vi "Configure Threshold Range.vi"(6 "Auto Threshold Range (T: Enable)":bool=TRUE, 7 "Range (10)":dbl=10.0, 8 "error in (no error)":errorcluster, 9 "Channel List(\"\")":string, 10 "Function (10:Frequency)":i32(ring)=10 items=["Frequency"=10, "Period"=11], 11 "VISA resource name":refnum<visa-resource-name>) -> (0 "error out":errorcluster, 3 "VISA resource name out":refnum<visa-resource-name>)   [LabVIEW 2015, in "Keithley DMM6500 DAQ6500 Series.lvlib"]
doc: "Configures frequency and period threshold settings."
uses:
  <instrlib>/Keithley DMM6500 DAQ6500 Series/Keithley DMM6500 DAQ6500 Series.lvlib
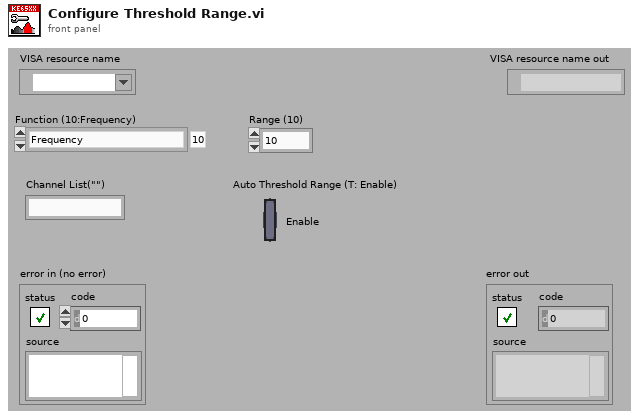
[diagram p1: front panel]
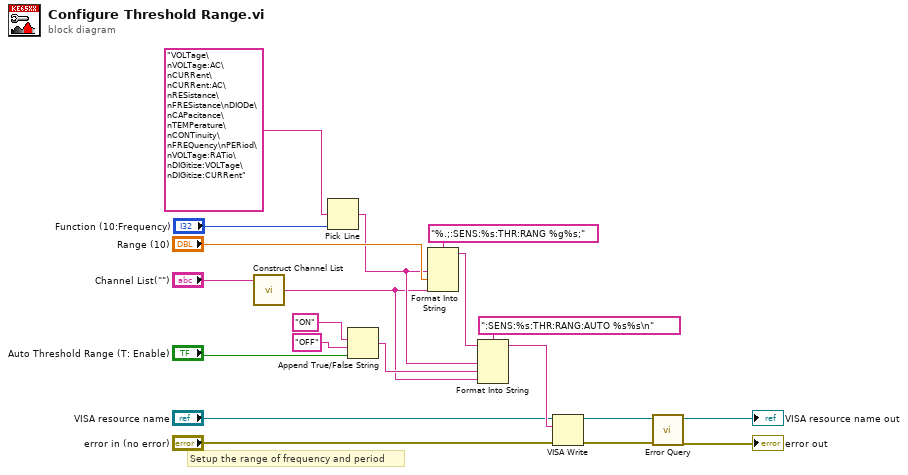
[diagram p0: block diagram]
diagram:
  # "Setup the range of frequency and period"
  n1 = call <instrlib>:"Construct Channel List.vi"("Channel List"="Channel List(\"\")") -> ("Channel List String"=w1:string)  [unwired: 2 in]
  n2 = Pick Line(multi-line string="VOLTage\nVOLTage:AC\nCURRent\nCURRent:AC\nRESistance\nFRESistance\nDIODe\nCAPacitance\nTEMPerature\nCONTinuity\nFREQuency\nPERiod\nVOLTage:RATio\nDIGitize:VOLTage\nDIGitize:CURRent" ("string (\"\")"), line index="Function (10:Frequency)") -> (output string=w3:string)  [unwired: 1 in]
  n3 = Append True/False String(1:"Auto Threshold Range (T: Enable)", 2:"OFF", 3:"ON") -> (0:w13:string)  [unwired: 1 in]
  n4 = Format Into String(format string="%.;:SENS:%s:THR:RANG %g%s;", w3, "Range (10)", w1) -> (resulting string=w15:string)  [unwired: 2 in, 1 out]
  n5 = Format Into String(format string=":SENS:%s:THR:RANG:AUTO %s%s\n", initial string=w15, w3, w13, w1) -> (resulting string=w12:string)  [unwired: 1 in, 1 out]
  n6 = VISA Write(VISA resource name="VISA resource name", write buffer=w12, error in (no error)="error in (no error)") -> (VISA resource name out=w9:refnum<visa-resource-name>, error out=w8:errorcluster)  [unwired: 1 out]
  n7 = call <instrlib>:"Error Query.vi"("error in (no error)"=w8, "VISA resource name"=w9) -> ("error out"=→"error out":errorcluster, "VISA resource name out"=→"VISA resource name out":refnum<visa-resource-name>)  [unwired: 6 in, 2 out]
